vi "Average2DArrayofSamples.vi"(2 "Sample Size":i32=3, 3 "Number of Samples":i32=2, 4 "2D Array of Samples":dbl[][](array[numeric])) -> (0 "Std Devs":dbl[][](array[numeric]), 1 "Averages":dbl[][](array[numeric]))   [LabVIEW 2016]
uses:
  <vilib>/Analysis/NI_AALBase.lvlib
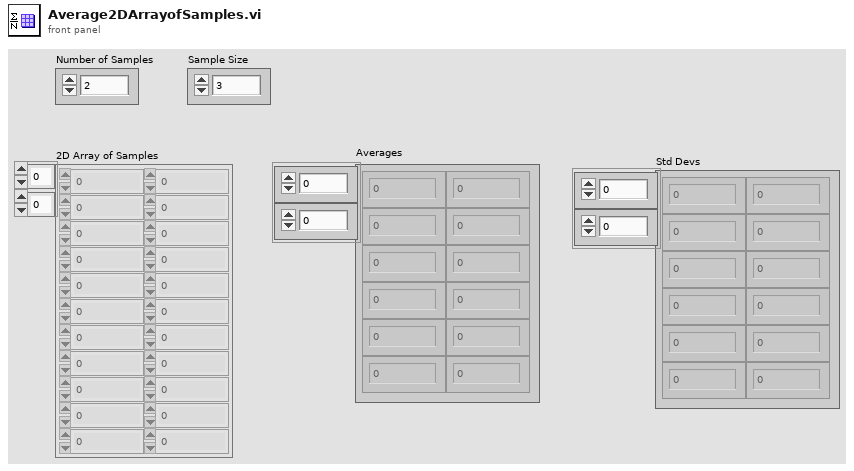
[diagram p1: front panel]
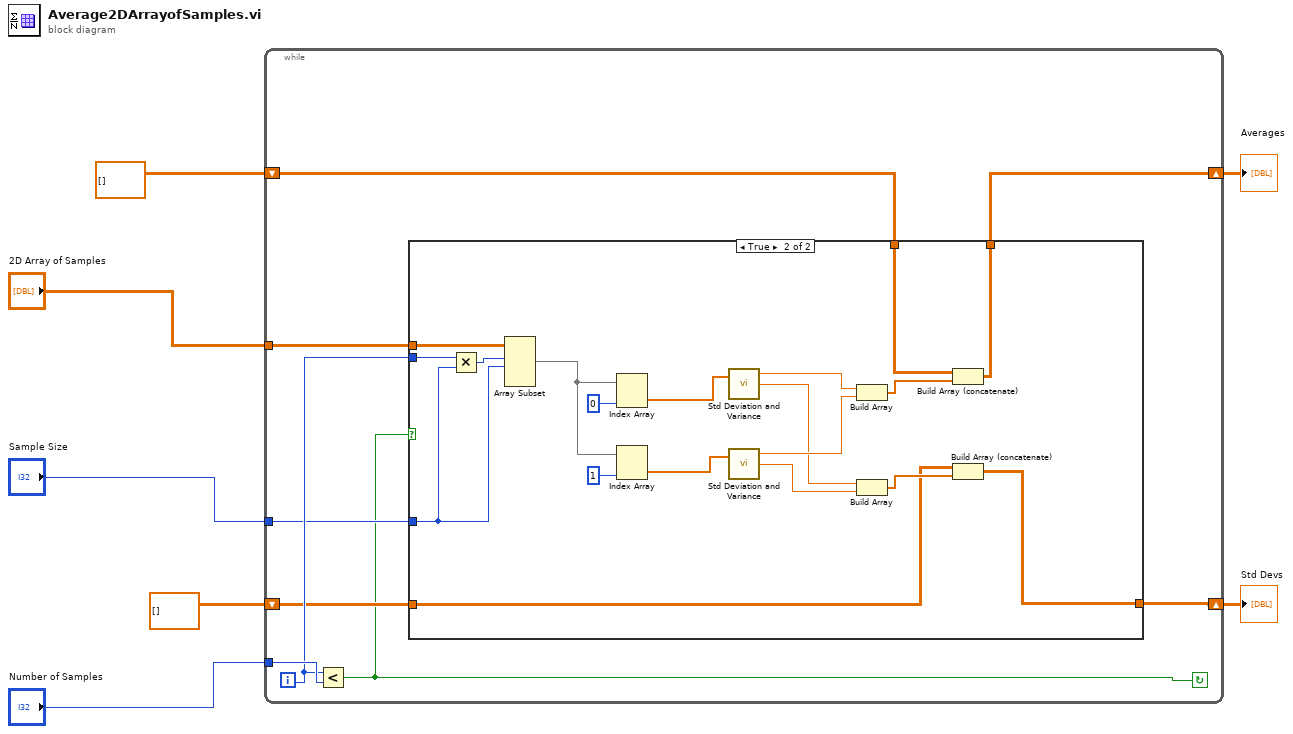
[diagram p0: block diagram]
diagram:
  n1 = while {
    tunnel: "Number of Samples" -> [w16]
    tunnel: "2D Array of Samples" -> [w15]
    tunnel: "Sample Size" -> [w13]
    shift-right: [w11] -> w2
    shift-left: dbl[][] [] -> [w12]
    shift-right: [w9] -> w1
    shift-left: dbl[][] [] -> [w10]
    i -> [w14]
    stop <- w8 continue-if-true
    n2 = Less?(x=w14, y=w16) -> (x < y?=w8:bool)
    n3 = case shown="True" w8 {
      tunnel: w15 -> [_ w37]
      tunnel: w14 -> [_ w35]
      tunnel: w13 -> [_ w34]
      tunnel: w12 -> [w18 w23]
      tunnel: [w18 w22] -> w11
      tunnel: w10 -> [w17 w20]
      tunnel: [w17 w19] -> w9
      frame False {
      }
      frame True {
        n4 = Multiply(x=w35, y=w34) -> (x*y=w36:i32)
        n5 = Array Subset(array=w37, index (row)=w36, length (row)=w34) -> (w31:dbl[][])  [unwired: 2 in]
        n6 = Index Array(array=w31, index (col)=0 ("disabled index (col)")) -> (element=w30:dbl[])  [unwired: 1 in]
        n7 = Index Array(array=w31, index (col)=1 ("disabled index (col)")) -> (element=w29:dbl[])  [unwired: 1 in]
        n8 = call <vilib>:"Std Deviation and Variance.vi"("X"=w30) -> ("mean"=w28:dbl, "standard deviation"=w26:dbl)  [unwired: 1 in, 1 out]
        n9 = call <vilib>:"Std Deviation and Variance.vi"("X"=w29) -> ("mean"=w27:dbl, "standard deviation"=w25:dbl)  [unwired: 1 in, 1 out]
        n10 = Build Array(w28, w27) -> (w24:dbl[])
        n11 = Build Array(w26, w25) -> (w21:dbl[])
        n12 = Build Array (concatenate)(w23, w24) -> (w22:dbl[][])
        n13 = Build Array (concatenate)(w20, w21) -> (w19:dbl[][])
      }
    }
  }
  "Averages" <- w2
  "Std Devs" <- w1
